vi "FPGAmain_5782_IQ_PID_Quench.vi"() -> ()   [LabVIEW 2018]
uses:
  FPGA/DataMode.ctl
  FPGA/Input_5782/5782_Fast_PID_states.ctl
  FPGA/Feed forward/FeedForwardState.ctl
  FPGA/Feed forward/FeedForwardProcessingState.ctl
  <vilib>/Platform/TimedLoop/XDataNode/timing_clust.ctl
  <vilib>/Platform/TimedLoop/XDataNode/nitl_modes.ctl
  <vilib>/Platform/TimedLoop/XDataNode/wakeup.ctl
  <vilib>/rvi/Emulation/niFpgaSctlEmulationGetInTimedLoop.vi
  <vilib>/rvi/Emulation/niFpgaEmulationReportErrorSimple.vi
  <vilib>/rvi/Emulation/niFpgaGetClockAttributes.vi
  <vilib>/rvi/Emulation/niFpgaCriticalErrorInLSC.vi
  <vilib>/rvi/Emulation/niFpgaProcessEmulError.vi
  <vilib>/rvi/Emulation/niFpgaEmulationIsFPGAContextNoSignature.vi
  <vilib>/rvi/errors/niFpgaSetErrorForExecOnDevCompSimple.vi
  <vilib>/rvi/eio/common/nirviEmuReportErrorAndStop.vi
  <vilib>/rvi/DataTransferAndStorage/Container/Common/niFpgaContainerGetUniqueNameForEmu.vi
  <vilib>/rvi/FIFO/Fifo_Resource/nirvififoEmulationSetSize.vi
  <vilib>/rvi/FIFO/Fifo_Resource/nirviFifoEmulationQueueMgr.vi
  <instcachedir>/0/nirviFifoEmulationQueueMgr_E5CAEC123FF24DC58D834DCA3CDAA9B5.lvgen/nirviFifoEmulationQueueMgr_E5CAEC123FF24DC58D834DCA3CDAA9B5_015.vi
  <vilib>/rvi/FIFO/Fifo_Resource/nirvififoEmulationDetermineInputValidOut.vi
  <vilib>/rvi/FIFO/Fifo_Resource/nirvififoEmulationCreateLock.vi
  <vilib>/rvi/FIFO/Fifo_Resource/nirvififoEmulationObtainLock.vi
  <vilib>/rvi/FIFO/Fifo_Resource/nirvififoEmulationReleaseLock.vi
  <vilib>/rvi/occurrence/nirviWaitOnOccurrenceBase.vi
  <vilib>/rvi/errors/nirviReportUnexpectedCaseInternalError.vi
  <vilib>/rvi/errors/nirviReportUnexpectedCaseInternalError (U32).vi
  <vilib>/rvi/Memory/Memory_Emulation/niFpgaMemoryEmulationCacheClearOnFirstRun.vi
  <vilib>/rvi/Memory/Memory_Emulation/nirvimemoryEmulationManagerCache_MakeExclusive.vi
  <vilib>/rvi/Memory/Memory_Emulation/niFpgaMemoryEmulationValidateCache.vi
  <vilib>/rvi/Memory/Memory_Emulation/nirvimemoryEmulationManagerCache_InsertValue.vi
  <vilib>/Utility/error.llb/Clear Errors.vi
  <vilib>/rvi/Memory/Memory_Emulation/nirvimemoryEmulationManagerCache_ReleaseExclusive.vi
  <vilib>/rvi/Memory/Memory_Emulation/nirvimemoryEmulationManagerCache_GetValue.vi
  <vilib>/rvi/Memory/Memory_Emulation/nirvimemoryEmulationManagerCache_SetValue.vi
  <vilib>/rvi/eio/common/nirviEmuTemplateMethod_errors.vi
  <instcachedir>/0/nirviFifoEmulationQueueMgr_E5CAEC123FF24DC58D834DCA3CDAA9B5.lvgen/nirviFifoEmulationQueueMgr_E5CAEC123FF24DC58D834DCA3CDAA9B5_018.vi
  <vilib>/rvi/interface/RandomDataEmulation/niFpgaRandomDataHandleErrors.vi
  <instcachedir>/0/nirviFifoEmulationQueueMgr_E5CAEC123FF24DC58D834DCA3CDAA9B5.lvgen/nirviFifoEmulationQueueMgr_E5CAEC123FF24DC58D834DCA3CDAA9B5_003.vi
  <instcachedir>/0/nirviFifoEmulationQueueMgr_E5CAEC123FF24DC58D834DCA3CDAA9B5.lvgen/nirviFifoEmulationQueueMgr_E5CAEC123FF24DC58D834DCA3CDAA9B5_017.vi
  <vilib>/rvi/interface/RandomDataEmulation/nirviRandomDataMultiElementFPGAFIFO.vi
  <instcachedir>/0/nirviRandomDataMultiElementFPGAFIFO_6740B454F3C245F78F76ED91F73FD8DB.lvgen/nirviRandomDataMultiElementFPGAFIFO_6740B454F3C245F78F76ED91F73FD8DB_000.vi
  <instrlib>/_niInstr/Basic Elements/v1/FPGA/Private/Count Down U8.vi
  <vilib>/rvi/Memory/Memory_Emulation/nirvimemoryFastEmulation.vi
  <vilib>/rvi/Memory/Memory_Emulation/nirvimemoryEmulation.vi
  <instcachedir>/0/nirviFifoEmulationQueueMgr_E5CAEC123FF24DC58D834DCA3CDAA9B5.lvgen/nirviFifoEmulationQueueMgr_E5CAEC123FF24DC58D834DCA3CDAA9B5_020.vi
  <vilib>/Platform/TimedLoop/XDataNode/XDataNode.xnode
  <vilib>/rvi/FXPMathLib/FxpInterpret/XNode/nifxpmath_Interpret.xnode
  <vilib>/rvi/DataTransferAndStorage/Container/XNode/niFpgaContainer.xnode
  <vilib>/rvi/FIFO/Fifo_Resource/nirvififoEmulationWrite.vi
  <vilib>/rvi/DataTransferAndStorage/Register/Emulation/niFpgaRegisterEmulation.vi
  <vilib>/eio/EIONode/EIONode.xnode
  <vilib>/rvi/FIFO/Fifo_Resource/nirvififoEmulationRead.vi
  <vilib>/rvi/interface/RandomDataEmulation/nirviRandomDataFpgaReadWriteTemplate.vi
  <vilib>/rvi/interface/RandomDataEmulation/nirviRandomDataFpgaMultiElementTemplate.vi
  <vilib>/Platform/TimedLoop/XDataNode/XDNodeRunTimeDep.lvlib
  <instrlib>/_niInstr/Basic Elements/v1/FPGA/niInstr Basic Elements v1 FPGA.lvlib
panel:
  out "TaM":fxp<+/-,32,13>
  out "Quench_Warning":bool
  out "Tau_set":fxp<+/-,32,13>
  in  "Ultra low speed transfer":bool
  out "5782 states":T1
  out "Read FF address":u32
  in  "Load FF":bool
  in  "Clear feedback buffers":bool
  in  "FF buffers manual":bool
  in  "Full speed transfer":bool
  in  "IO Module\\AO Data Sync":bool=TRUE
  in  "IO Module\\SPI Write Data":u16
  out "IO Module\\SPI Read Data":u8
  in  "IO Module\\SPI Read":bool
  in  "IO Module\\SPI Write":bool
  in  "IO Module\\SPI Address":u16
  in  "IO Module\\SPI Device":u8
  out "IO Module\\SPI Idle":bool
  in  "AM phase":fxp<+,64,64>
  in  "User Command Commit":bool
  in  "User Command":u8
  out "User Command Idle":bool
  out "User Command Status":u8
  in  "User Data 0":u8
  in  "User Data 1":u8
  out "PLL Locked":bool
  out "User Error":bool
  out "Configured?":bool
  in  "Continuous":bool
  in  "Record length":u16=4000 caption="Samples Per Trigger" min=1 step=1
  in  "Trigger Acquisition":bool
  out "IO Module\\Trigger Input":bool
  in  "Acquisition running":bool
  in  "Phase output":fxp<+,64,64>[](array[numeric])=[0.0, 0.0, 0.0, 0.0]
  in  "Simulated phase":fxp<+,64,64>[](array[numeric])=[0.0, 0.0]
  in  "Mode":T2
  in  "Phase input":fxp<+,64,64>[](array[numeric])=[0.0, 0.0, 0.0, 0.0, 0.0, 0.0, 0.0, 0.0, 0.0, 0.0, 0.0, 0.0, 0.0, 0.0, 0.0, 0.0]
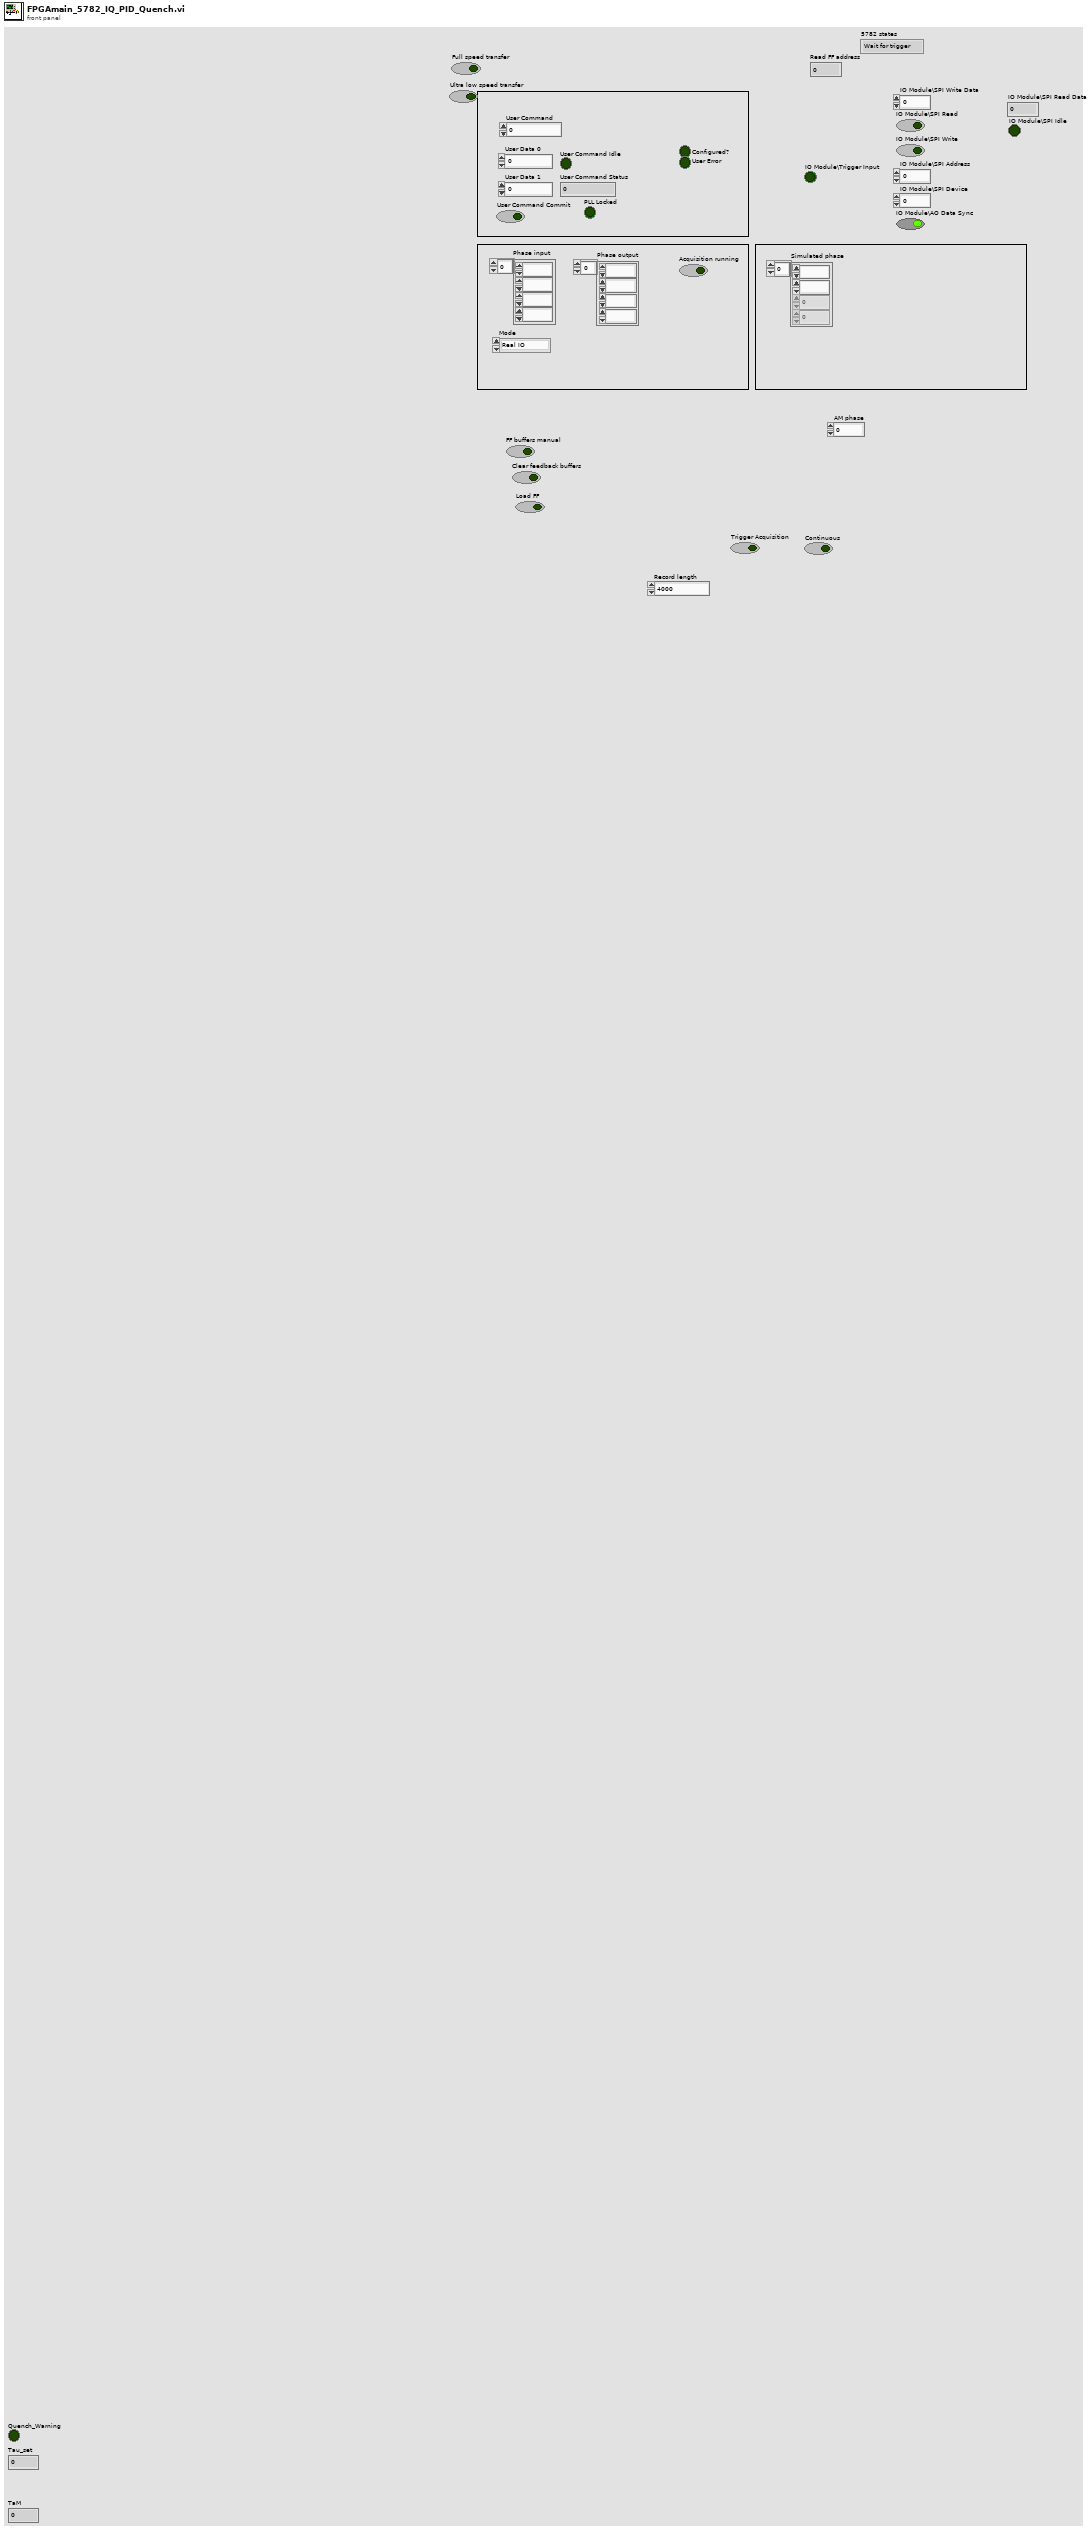
[diagram p1: front panel]
types:
  T1 = typedef "5782_Fast_PID_states.ctl" = enum8{"Wait for trigger", "Acquisition", "Send record length", "Wait for output", "Quiet period"}
  T2 = typedef "DataMode.ctl" = enum16{"Real IO", "Simulated"}
  T3 = typedef "FeedForwardProcessingState.ctl" = enum16{"Wait for trigger", "Processing", "Filtering", "Wait for reset"}
  T4 = typedef "FeedForwardState.ctl" = enum16{"Idle", "Wait for trigger", "Read FF", "Clear FF", "Wait for reset"}
  T5 = typedef "XDNodeRunTimeDep.lvlib/timing_clust.ctl" = cluster{"Expected End [f-1]":u64, "Actual End [f-1]":u64, "Finished Late? [f-1]":bool, "Expected End [i-1]":u64, "Actual End [i-1]":u64, "Finished Late? [i-1]":bool, "Expected Start [i]":u64, "Actual Start [i]":u64, "Expected Start [f]":u64, "Actual Start [f]":u64, "Source Name":string, "Structure Name":string, "Period":i64, "Deadline":i64, "Offset":i64, "Start":i64, "Priority":i32, "Timeout":i32, "Mode":T6, "Wakeup Reason":T7, "Error":errorcluster, "Source Type":string, "Secondary Source Type":string, "Global End Time":u64, "Global Start Time":u64, "Frame Duration":u64, "Iteration Duration":u64, "Assigned CPU":i32, "I/O Scan Engine Mode":u32}
  T6 = typedef "XDNodeRunTimeDep.lvlib/nitl_modes.ctl" = enum32{"No Change", "Process missed periods, maintain original phase", "Discard missed periods, maintain original phase", "Process missed periods, ignore original phase", "Discard missed periods, ignore original phase"}
  T7 = typedef "XDNodeRunTimeDep.lvlib/wakeup.ctl" = enum32{"Normal", "Aborted", "Asynchronous wakeup", "Timing source error", "Timed loop error", "Timeout"}
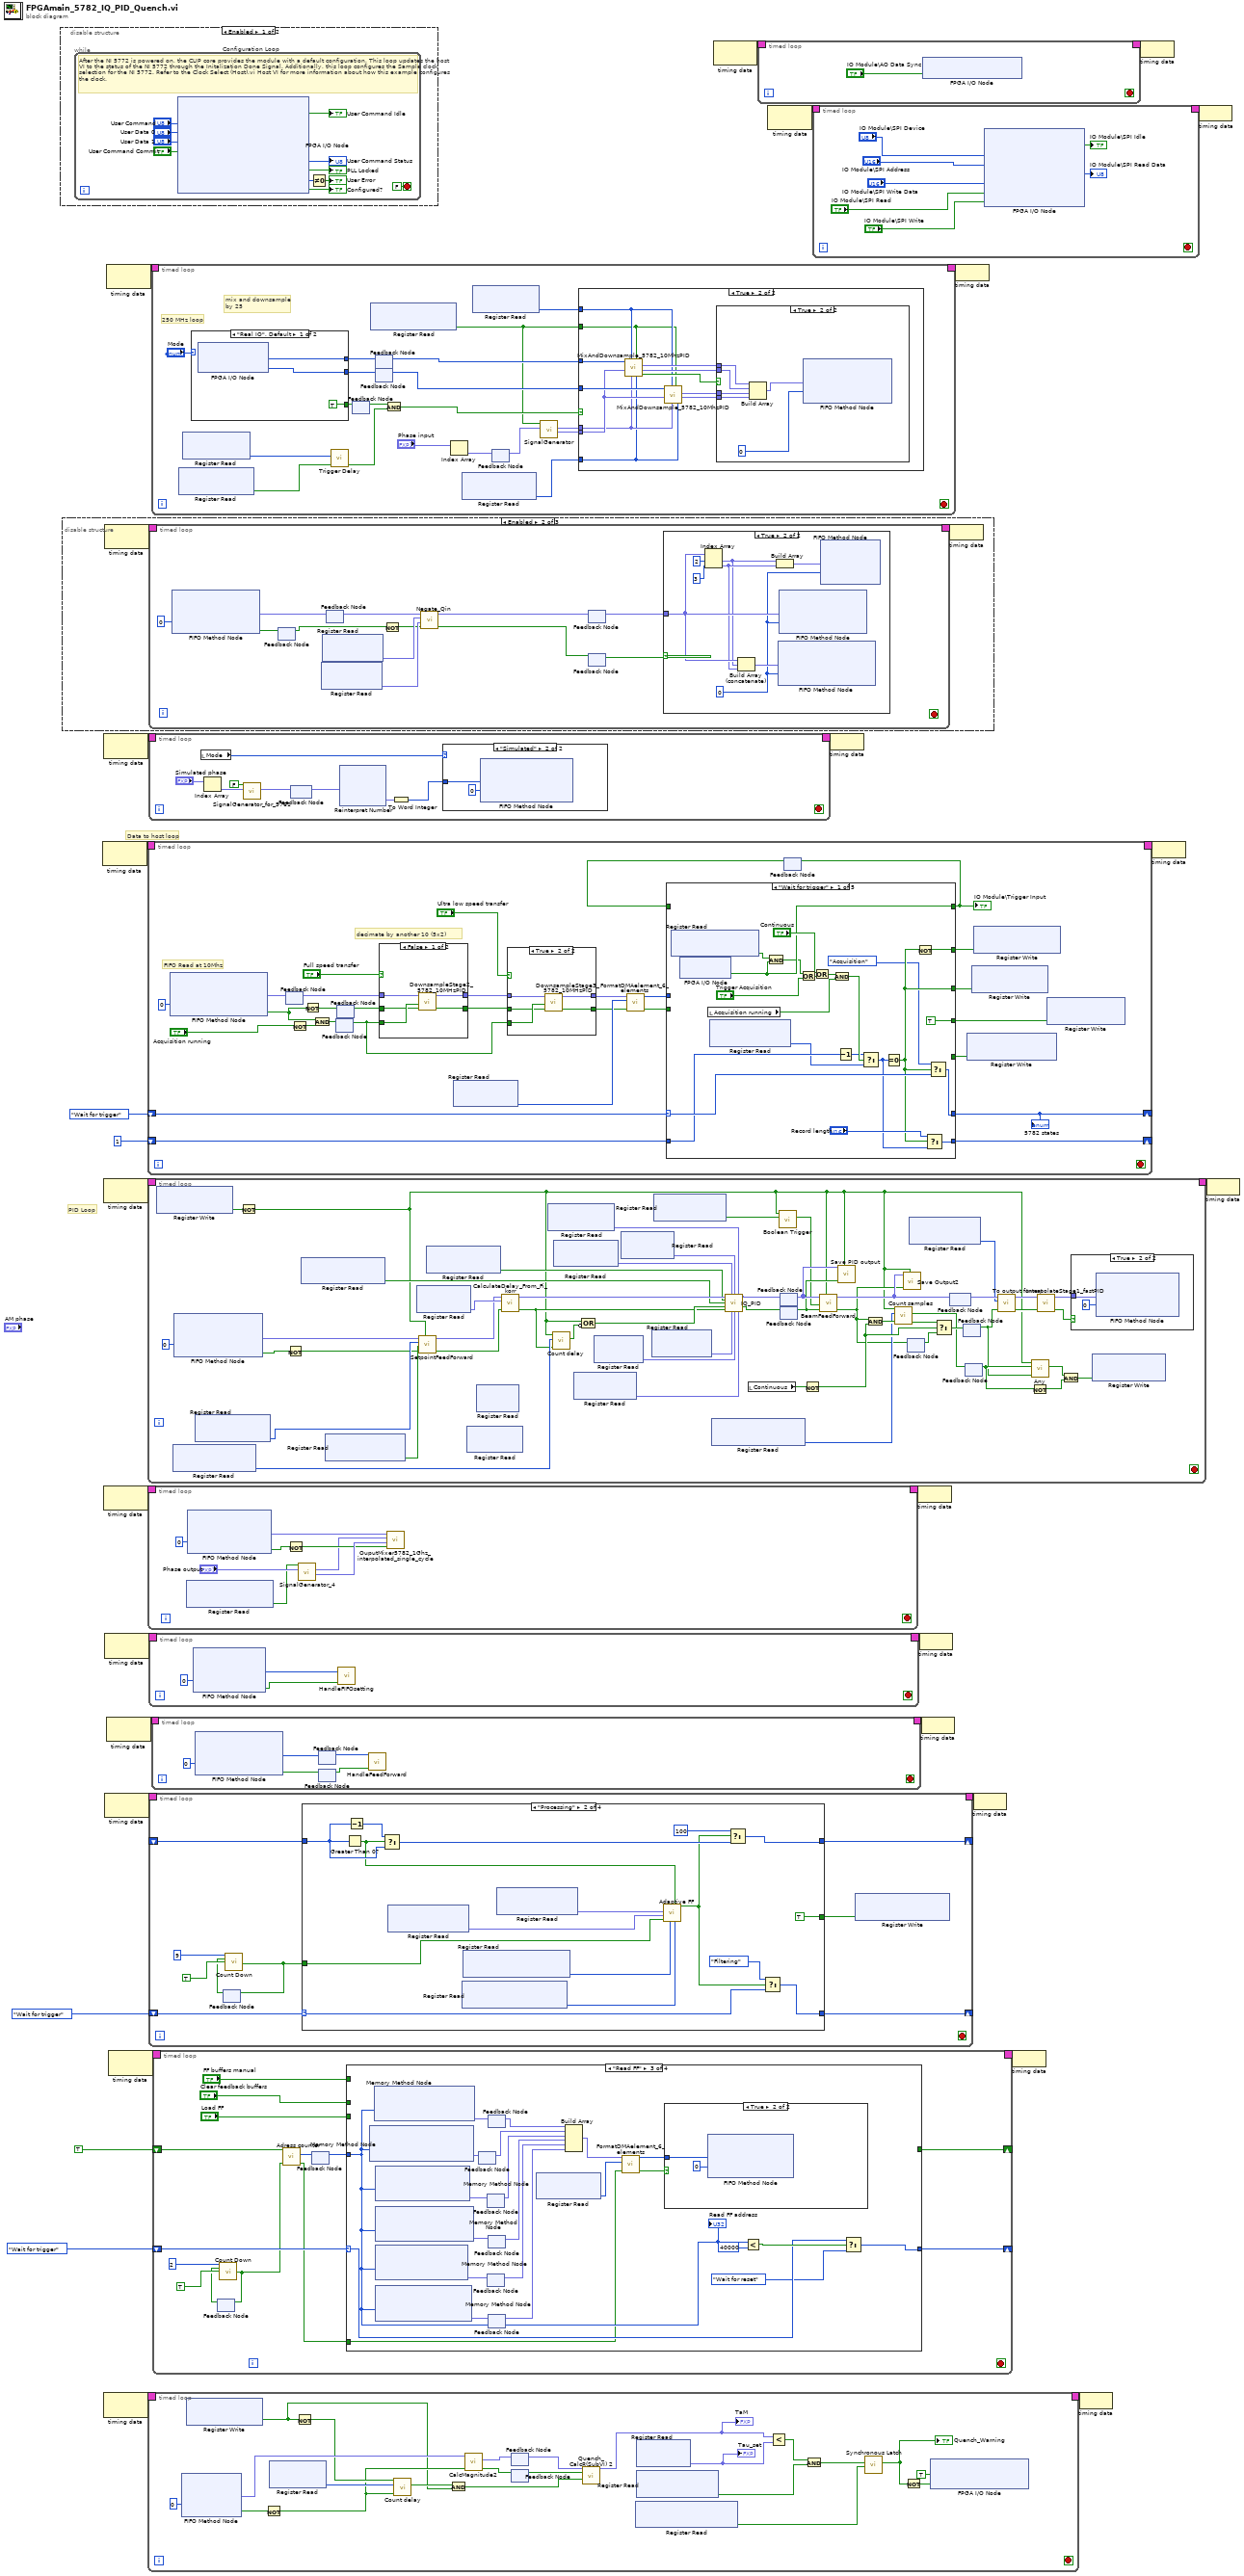
[diagram p0: block diagram]
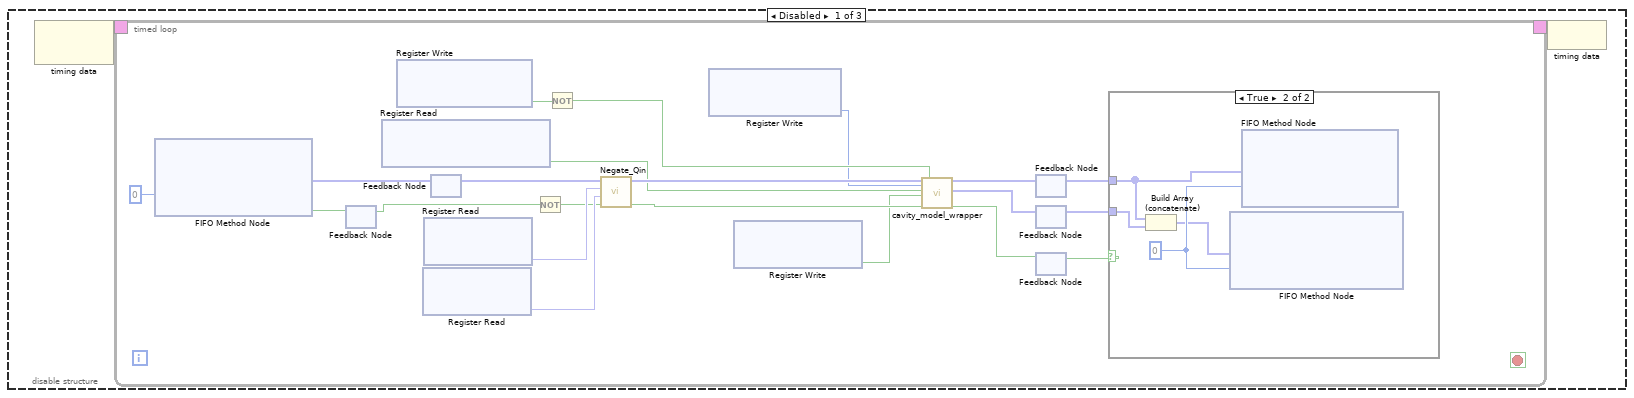
[diagram p2: hidden frame]
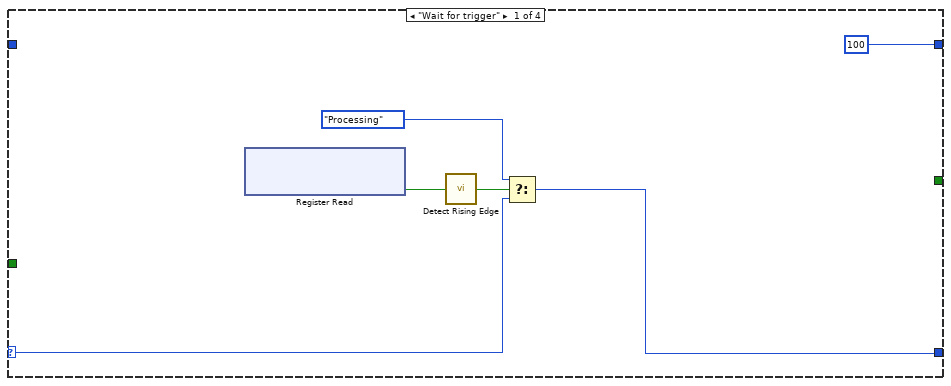
[diagram p6: hidden frame]
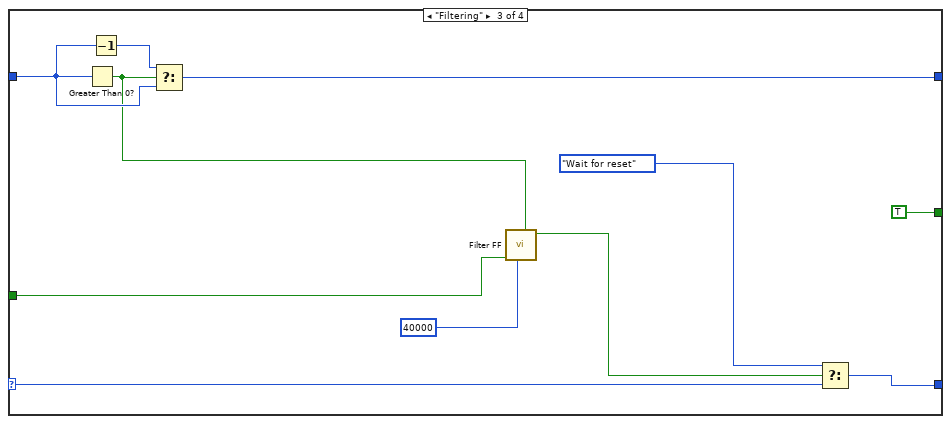
[diagram p7: hidden frame]
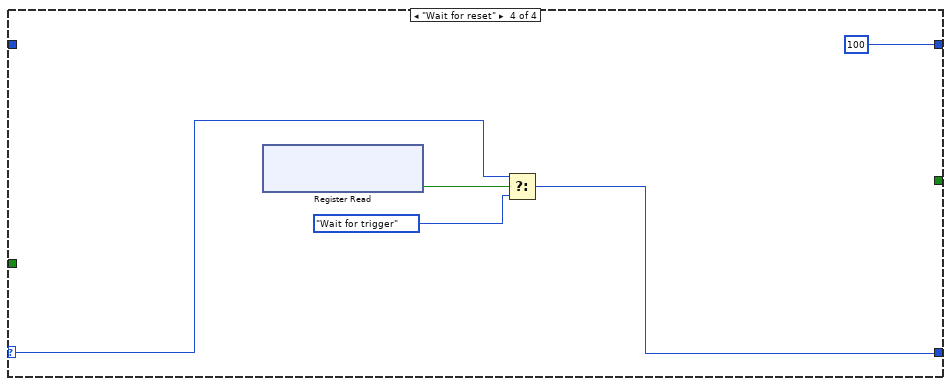
[diagram p8: hidden frame]
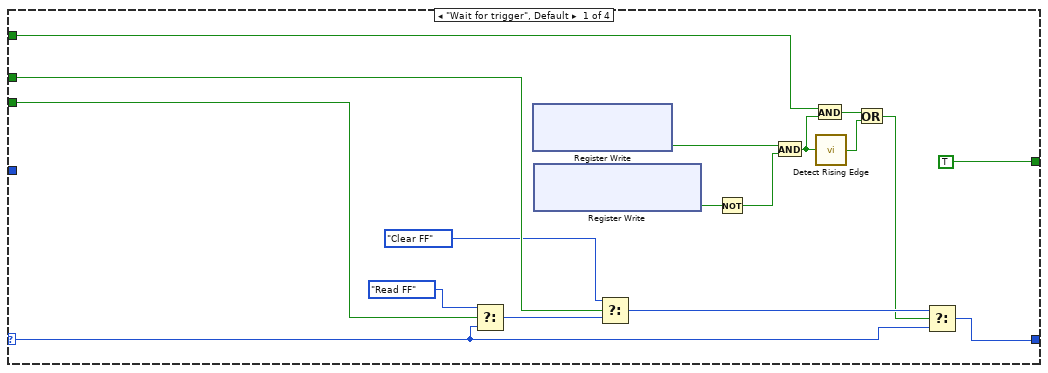
[diagram p9: hidden frame]
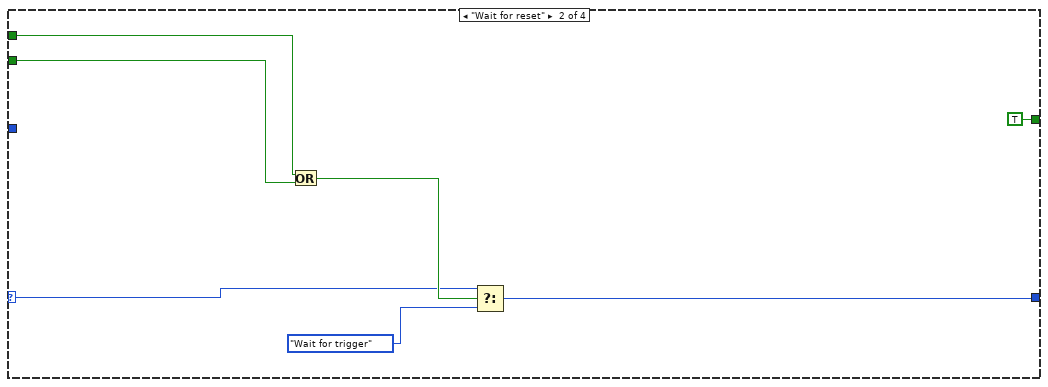
[diagram p10: hidden frame]
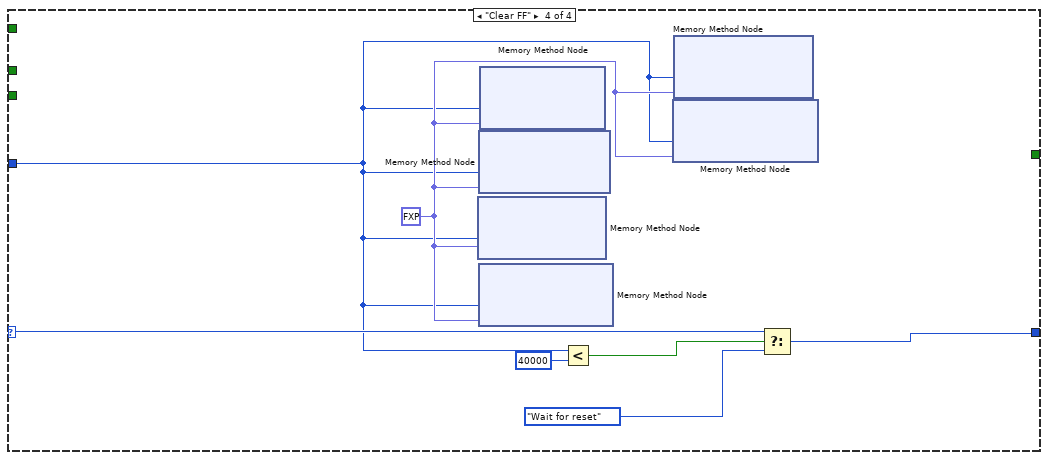
[diagram p12: hidden frame]
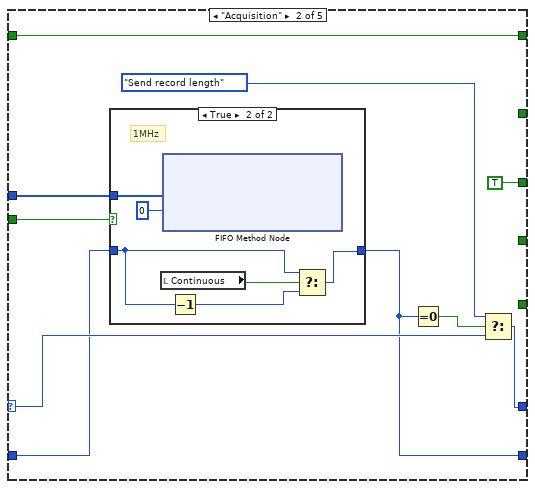
[diagram p15: hidden frame]
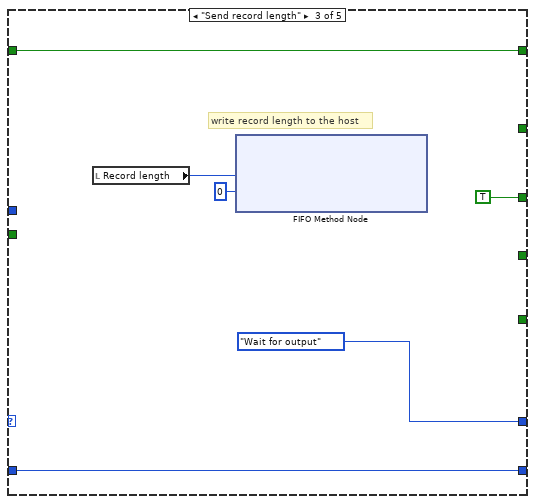
[diagram p17: hidden frame]
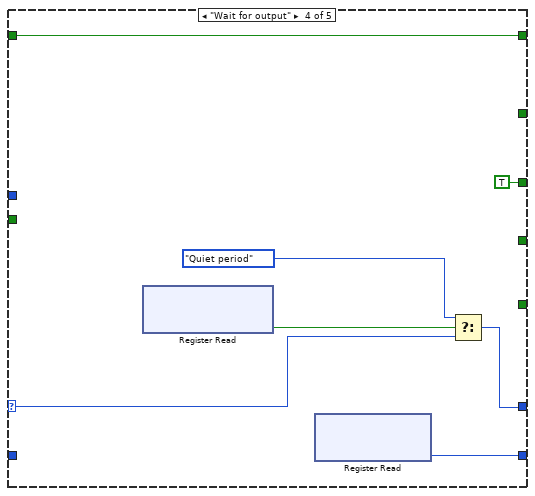
[diagram p18: hidden frame]
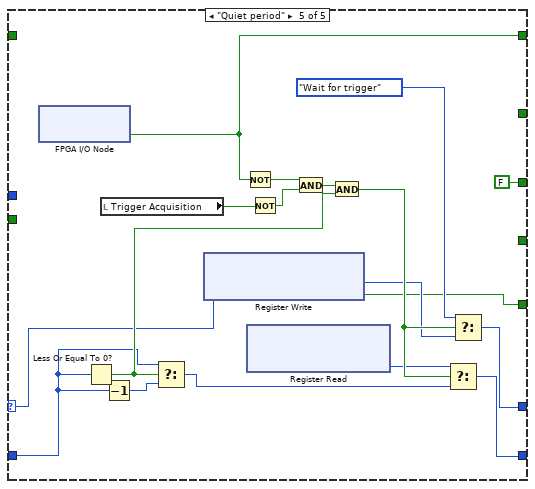
[diagram p19: hidden frame]
diagram:
  # "PID Loop"
  # "Data to host loop"
  n1 = disable-structure shown="Enabled" {
    frame Enabled {
      n2 = while "Configuration Loop" {
        stop <- FALSE stop-if-true
        # "After the NI 5772 is powered on, the CLIP core provides the module with a default configuration. This loop updates the host VI to the status of the NI 5772 through the Initalization Done Signal. Additionally, this loop configures the Sample clock selection for the NI 5772. Refer to the Clock Select (Host).vi Host VI for more information about how this example configures the clock."
        n3 = xnode "FPGA I/O Node"("IO Module\\User Command"="User Command", "IO Module\\User Data 0"="User Data 0", "IO Module\\User Data 1"="User Data 1", "IO Module\\User Command Commit"="User Command Commit") -> ("IO Module\\User Command Idle"=→"User Command Idle":bool, "IO Module\\User Command Status"=→"User Command Status":u8, "IO Module\\PLL Locked"=→"PLL Locked":bool, "IO Module\\User Error"=w35:u8, "IO Module\\Initialization Done"=→"Configured?":bool)  [unwired: 9 in, 9 out]
        n4 = Not Equal To 0?(x=w35) -> (x != 0?=→"User Error":bool)
      }
    }
    frame Disabled {
    }
  }
  n5 = disable-structure shown="Enabled" {
    frame Disabled {
      n6 = node-c288() -> (w42:T5)  [unwired: 1 in]
      n7 = timed-loop {
        timing: w42 -> [_]
        timing-out: [_] -> w41
        stop <- _ stop-if-true
        n8 = xnode ("FIFO Method Node")("Timeout"=0) -> ("Element"=w49:fxp<+/-,32,14>[], "Timed Out?"=w48:bool)  [unwired: 1 in, 1 out]
        n9 = feedback #1() -> (w46:bool)  [unwired: 1 in]
        n10 = feedback-in #1(w48) -> ()
        n11 = xnode ("Register Read")() -> ("Data"=w57:bool)  [unwired: 1 in, 1 out]
        n12 = xnode ("Register Write")() -> ("Data"=w56:bool)  [unwired: 1 in, 1 out]
        n13 = xnode ("Register Read")() -> ("Data"=w62:fxp<+/-,32,14>)  [unwired: 1 in, 1 out]
        n14 = xnode ("Register Read")() -> ("Data"=w63:fxp<+/-,32,14>)  [unwired: 1 in, 1 out]
        n15 = feedback #2() -> (w47:fxp<+/-,32,14>[])  [unwired: 1 in]
        n16 = feedback-in #2(w49) -> ()
        n17 = Not(x=w46) -> (.not. x?=w61:bool)
        n18 = Not(x=w56) -> (.not. x?=w58:bool)
        n19 = call "Negate_Qin.vi"("valid in"=w61, "DC offset chan 1"=w62, "DC offset chan 0"=w63, "Data in"=w47) -> ("valid out"=w59:bool, "Data out"=w60:fxp<+/-,32,14>[])  [unwired: 6 in]
        n20 = xnode "Register Write"() -> ("Data"=w43:enum16{"Off", "On - Ch 0", "On - Ch 1"})  [unwired: 1 in, 1 out]
        n21 = xnode "Register Write"() -> ("Data"=w44:bool)  [unwired: 1 in, 1 out]
        n22 = call "cavity_model_wrapper.vi"("Data in"=w60, "Piezo setting"=w43, "enabled"=w57, "virtual cavity"=w44, "input valid"=w59, "reset"=w58) -> ("Data out"=w55:fxp<+/-,32,14>[], "Ai1 out"=w51:fxp<+/-,32,14>[], "output valid"=w53:bool)  [unwired: 11 in]
        n23 = feedback #3() -> (w54:fxp<+/-,32,14>[])  [unwired: 1 in]
        n24 = feedback-in #3(w55) -> ()
        n25 = feedback #4() -> (w50:fxp<+/-,32,14>[])  [unwired: 1 in]
        n26 = feedback-in #4(w51) -> ()
        n27 = feedback #5() -> (w52:bool)  [unwired: 1 in]
        n28 = feedback-in #5(w53) -> ()
        n29 = case shown="True" w52 {
          tunnel: w54 -> [_ w66]
          tunnel: w50 -> [_ w65]
          frame False {
          }
          frame True {
            w67 = 0 ("Timeout")
            n30 = Build Array (concatenate)(w66, w65) -> (w64:fxp<+/-,32,14>[])
            n31 = xnode ("FIFO Method Node")("Element"=w64, "Timeout"=w67) -> ()  [unwired: 1 in, 2 out]
            n32 = xnode ("FIFO Method Node")("Element"=w66, "Timeout"=w67) -> ()  [unwired: 1 in, 2 out]
          }
        }
      }
      n33 = node-c288(w41) -> ()
    }
    frame Enabled {
      n34 = node-c288() -> (w73:T5)  [unwired: 1 in]
      n35 = timed-loop {
        timing: w73 -> [_]
        timing-out: [_] -> w72
        stop <- _ stop-if-true
        n36 = xnode ("FIFO Method Node")("Timeout"=0) -> ("Element"=w80:fxp<+/-,32,14>[], "Timed Out?"=w79:bool)  [unwired: 1 in, 1 out]
        n37 = feedback #6() -> (w77:bool)  [unwired: 1 in]
        n38 = feedback-in #6(w79) -> ()
        n39 = xnode ("Register Read")() -> ("Data"=w84:fxp<+/-,32,14>)  [unwired: 1 in, 1 out]
        n40 = xnode ("Register Read")() -> ("Data"=w85:fxp<+/-,32,14>)  [unwired: 1 in, 1 out]
        n41 = feedback #7() -> (w78:fxp<+/-,32,14>[])  [unwired: 1 in]
        n42 = feedback-in #7(w80) -> ()
        n43 = Not(x=w77) -> (.not. x?=w83:bool)
        n44 = call "Negate_Qin.vi"("valid in"=w83, "DC offset chan 1"=w84, "DC offset chan 0"=w85, "Data in"=w78) -> ("valid out"=w74:bool, "Data out"=w75:fxp<+/-,32,14>[])  [unwired: 6 in]
        n45 = feedback #8() -> (w82:fxp<+/-,32,14>[])  [unwired: 1 in]
        n46 = feedback-in #8(w75) -> ()
        n47 = feedback #9() -> (w81:bool)  [unwired: 1 in]
        n48 = feedback-in #9(w74) -> ()
        n49 = case shown="True" w81 {
          tunnel: w82 -> [_ w91]
          frame False {
          }
          frame True {
            w88 = 0 ("Timeout")
            n50 = Index Array(array=w91, index #1=2 ("index"), index #2=3 ("index")) -> (element #1=w86:fxp<+/-,32,14>, element #2=w87:fxp<+/-,32,14>)
            n51 = Build Array (concatenate)(w91, w86, w87) -> (w93:fxp<+/-,32,14>[])
            n52 = Build Array(w86, w87) -> (w92:fxp<+/-,32,14>[])
            n53 = xnode ("FIFO Method Node")("Element"=w93, "Timeout"=w88) -> ()  [unwired: 1 in, 2 out]
            n54 = xnode ("FIFO Method Node")("Element"=w91, "Timeout"=w88) -> ()  [unwired: 1 in, 2 out]
            n55 = xnode ("FIFO Method Node")("Element"=w92, "Timeout"=w88) -> ()  [unwired: 1 in, 2 out]
          }
        }
      }
      n56 = node-c288(w72) -> ()
    }
    frame Disabled {
    }
  }
  n57 = node-c288() -> (w14:T5)  [unwired: 1 in]
  n58 = node-c288() -> (w16:T5)  [unwired: 1 in]
  n59 = node-c288() -> (w22:T5)  [unwired: 1 in]
  n60 = node-c288() -> (w2:T5)  [unwired: 1 in]
  n61 = node-c288() -> (w29:T5)  [unwired: 1 in]
  n62 = node-c288() -> (w24:T5)  [unwired: 1 in]
  n63 = node-c288() -> (w5:T5)  [unwired: 1 in]
  n64 = node-c288() -> (w27:T5)  [unwired: 1 in]
  n65 = node-c288() -> (w11:T5)  [unwired: 1 in]
  n66 = node-c288() -> (w9:T5)  [unwired: 1 in]
  n67 = timed-loop {
    timing: w14 -> [_]
    timing-out: [_] -> w13
    shift-right: [w124] -> _
    shift-left: 5782_Fast_PID_states."Wait for trigger" ("5782 states") -> [w126]
    shift-right: [w123] -> _
    shift-left: u16 1 ("trigger samples") -> [w125]
    stop <- _ stop-if-true
    # "FIFO Read at 10Mhz"
    # "decimate by another 10 (5x2)"
    n68 = xnode ("FIFO Method Node")("Timeout"=0) -> ("Element"=w106:fxp<+/-,32,14>[], "Timed Out?"=w105:bool)  [unwired: 1 in, 1 out]
    n69 = feedback #10() -> (w107:fxp<+/-,32,14>[])  [unwired: 1 in]
    n70 = feedback-in #10(w106) -> ()
    n71 = Not(x="Acquisition running") -> (.not. x?=w112:bool)
    n72 = Not(x=w105) -> (.not. x?=w110:bool)
    n73 = And(x=w105, y=w112) -> (x .and. y?=w109:bool)
    n74 = feedback #11() -> (w102:bool)  [unwired: 1 in]
    n75 = feedback-in #11(w109) -> ()
    n76 = feedback #12() -> (w111:bool)  [unwired: 1 in]
    n77 = feedback-in #12(w110) -> ()
    n78 = case shown="False" "Full speed transfer" {
      tunnel: [w138 w140] -> w100
      tunnel: [w137 w139] -> w101
      tunnel: w107 -> [w136 w140]
      tunnel: w102 -> [w135 _]
      tunnel: w111 -> [w134 w139]
      frame False {
        n79 = call "DownsampleStage2_5782_10MHzPID.vi"("valid in"=w134, "reset"=w135, "Data in"=w136) -> ("valid out"=w137:bool, "data out"=w138:fxp<+/-,32,14>[])  [unwired: 7 in]
      }
      frame True {
      }
    }
    n80 = xnode ("Register Read")() -> ("Data"=w116:u16)  [unwired: 1 in, 1 out]
    n81 = case shown="True" "Ultra low speed transfer" {
      tunnel: [w128 w132] -> w98
      tunnel: [w127 w131] -> w99
      tunnel: w100 -> [w128 w133]
      tunnel: w102 -> [_ w130]
      tunnel: w101 -> [w127 w129]
      frame False {
      }
      frame True {
        n82 = call "DownsampleStage3_5782_10MHzPID.vi"("valid in"=w129, "reset"=w130, "Data in"=w133) -> ("valid out"=w131:bool, "data out"=w132:fxp<+/-,32,14>[])  [unwired: 7 in]
      }
    }
    n83 = call "FormatDMAelement_6_elements.vi"("valid in"=w99, "factor"=w116, "Data in"=w98) -> ("valid out"=w119:bool, "Values"=w118:u64[])  [unwired: 7 in]
    n84 = feedback #13() -> (w121:bool)  [unwired: 1 in]
    n85 = case shown="\"Wait for trigger\"" w126 {
      selector: w126 -> [w161 w171 _ w189 w196]
      tunnel: w125 -> [w152 w168 w179 _ w197]
      tunnel: [w160 w170 5782_Fast_PID_states."Wait for output" ("5782 states") w191 w207] -> w124
      tunnel: [w159 w165 w179 w187 w208] -> w123
      tunnel: w118 -> [_ w166 _ _ _]
      tunnel: w119 -> [_ w167 _ _ _]
      tunnel: [w147 TRUE TRUE ("5782 triggered") TRUE ("5782 triggered") FALSE ("5782 triggered")] -> w122
      tunnel: [w142 w164 w181 w186 w192] -> w120
      tunnel: w121 -> [_ w164 w181 w186 _]
      tunnel: [w146 _ _ _ _] -> w117
      tunnel: [TRUE _ _ _ _] -> w115
      tunnel: [_ _ _ _ w194] -> w114
      frame "Wait for trigger" {
        n86 = xnode ("Register Read")() -> ("Data"=w143:bool)  [unwired: 1 in, 1 out]
        n87 = xnode "FPGA I/O Node"() -> ("PXI_Trig0"=w142:bool)  [unwired: 1 in, 1 out]
        n88 = local read "Acquisition running"() -> (w155:bool)
        n89 = xnode ("Register Read")() -> ("Data"=w148:u16)  [unwired: 1 in, 1 out]
        n90 = And(x=w143, y=w142) -> (x .and. y?=w141:bool)
        n91 = Or(x=w141, y="Trigger Acquisition") -> (x .or. y?=w151:bool)
        n92 = Or(x="Continuous", y=w151) -> (x .or. y?=w149:bool)
        n93 = And(x=w149, y=w155) -> (x .and. y?=w156:bool)
        n94 = Decrement(x=w152) -> (x-1=w153:u16)
        n95 = Select(t=w153, s=w156, f=w148) -> (s? t:f=w154:u16)
        n96 = Equal To 0?(x=w154) -> (x = 0?=w147:bool)
        n97 = Not(x=w147) -> (.not. x?=w146:bool)
        n98 = Select(t="Record length", s=w147, f=w154) -> (s? t:f=w159:u16)
        n99 = Select(t=5782_Fast_PID_states."Acquisition" ("5782 states"), s=w147, f=w161) -> (s? t:f=w160:T1)
      }
      frame "Acquisition" {
        n100 = case shown="True" w167 {
          tunnel: w166 -> [_ w178]
          tunnel: [w172 w175] -> w165
          tunnel: w168 -> [w172 w173]
          frame False {
          }
          frame True {
            # "1MHz"
            n101 = local read "Continuous"() -> (w176:bool)
            n102 = xnode ("FIFO Method Node")("Element"=w178, "Timeout"=0) -> ()  [unwired: 1 in, 2 out]
            n103 = Decrement(x=w173) -> (x-1=w174:u16)
            n104 = Select(t=w173, s=w176, f=w174) -> (s? t:f=w175:u16)
          }
        }
        n105 = Equal To 0?(x=w165) -> (x = 0?=w169:bool)
        n106 = Select(t=5782_Fast_PID_states."Send record length" ("5782 states"), s=w169, f=w171) -> (s? t:f=w170:T1)
      }
      frame "Send record length" {
        # "write record length to the host"
        n107 = local read "Record length"() -> (w183:u16)
        n108 = xnode ("FIFO Method Node")("Element"=w183, "Timeout"=0) -> ()  [unwired: 1 in, 2 out]
      }
      frame "Wait for output" {
        n109 = xnode ("Register Read")() -> ("Data"=w185:bool)  [unwired: 1 in, 1 out]
        n110 = xnode ("Register Read")() -> ("Data"=w187:u16)  [unwired: 1 in, 1 out]
        n111 = Select(t=5782_Fast_PID_states."Quiet period" ("5782 states"), s=w185, f=w189) -> (s? t:f=w191:T1)
      }
      frame "Quiet period" {
        n112 = xnode "FPGA I/O Node"() -> ("PXI_Trig0"=w192:bool)  [unwired: 1 in, 1 out]
        n113 = Less Or Equal To 0?(x=w197) -> (x <= 0?=w200:bool)
        n114 = local read "Trigger Acquisition"() -> (w205:bool)
        n115 = Decrement(x=w197) -> (x-1=w201:u16)
        n116 = Select(t=w197, s=w200, f=w201) -> (s? t:f=w199:u16)
        n117 = xnode ("Register Write")() -> ("Data"=w194:bool)  [unwired: 1 in, 1 out]
        n118 = Not(x=w192) -> (.not. x?=w193:bool)
        n119 = xnode ("Register Read")() -> ("Data"=w198:u16)  [unwired: 1 in, 1 out]
        n120 = Not(x=w205) -> (.not. x?=w204:bool)
        n121 = And(x=w193, y=w204) -> (x .and. y?=w203:bool)
        n122 = And(x=w203, y=w200) -> (x .and. y?=w206:bool)
        n123 = Select(t=w198, s=w206, f=w199) -> (s? t:f=w208:u16)
        n124 = Select(t=5782_Fast_PID_states."Wait for trigger" ("5782 states"), s=w206, f=w196) -> (s? t:f=w207:T1)
      }
    }
    "IO Module\\Trigger Input" <- w120
    "5782 states" <- w124
    n125 = feedback-in #13(w120) -> ()
    n126 = xnode ("Register Write")("Data"=w114) -> ()  [unwired: 1 in, 1 out]
    n127 = xnode ("Register Write")("Data"=w122) -> ()  [unwired: 1 in, 1 out]
    n128 = xnode ("Register Write")("Data"=w117) -> ()  [unwired: 1 in, 1 out]
    n129 = xnode ("Register Write")("Data"=w115) -> ()  [unwired: 1 in, 1 out]
  }
  n130 = timed-loop {
    timing: w16 -> [_]
    timing-out: [_] -> w15
    stop <- _ stop-if-true
    n131 = xnode ("Register Write")() -> ("Data"=w259:bool)  [unwired: 1 in, 1 out]
    n132 = xnode ("Register Read")() -> ("Data"=w255:u32)  [unwired: 1 in, 1 out]
    n133 = xnode ("FIFO Method Node")("Timeout"=0) -> ("Element"=w253:fxp<+/-,32,14>[], "Timed Out?"=w260:bool)  [unwired: 1 in, 1 out]
    n134 = xnode ("Register Read")() -> ("Data"=w254:u32)  [unwired: 1 in, 1 out]
    n135 = Not(x=w259) -> (.not. x?=w213:bool)
    n136 = Not(x=w260) -> (.not. x?=w252:bool)
    n137 = xnode ("Register Read")() -> ("Data"=w239:bool)  [unwired: 1 in, 1 out]
    n138 = xnode ("Register Read")() -> ("Data"=w258:bool)  [unwired: 1 in, 1 out]
    n139 = xnode ("Register Read")() -> ("Data"=w251:fxp<+/-,32,4>)  [unwired: 1 in, 1 out]
    n140 = call "SetpointFeedForward.vi"("Reset"=w213, "input valid"=w252, "setpoint enabled"=w258, "Samples to skip"=w254, "Data in"=w253) -> ("output valid"=w250:bool, "Data out"=w249:fxp<+/-,32,14>[])  [unwired: 5 in]
    n141 = xnode ("Register Read")() -> ("Data"=w247:bool)  [unwired: 1 in, 1 out]
    n142 = xnode ("Register Read")() -> ()  [unwired: 1 in, 2 out]
    n143 = xnode ("Register Read")() -> ()  [unwired: 1 in, 2 out]
    n144 = call "CalculateDelay_From_Fi_korr.vi"("input valid"=w250, "fi_korr"=w251, "Data in"=w249) -> ("output valid"=w240:bool, "Data out"=w248:fxp<+/-,32,14>[])  [unwired: 7 in]
    n145 = xnode ("Register Read")() -> ("Data"=w242:fxp<+/-,32,6>)  [unwired: 1 in, 1 out]
    n146 = call "Count delay.vi"("input valid"=w240, "Count to skip"=w255, "Reset"=w213) -> ("count done?"=w256:bool)  [unwired: 7 in, 1 out]
    n147 = xnode ("Register Read")() -> ("Data"=w246:fxp<+/-,32,6>)  [unwired: 1 in, 1 out]
    n148 = xnode ("Register Read")() -> ("Data"=w236:fxp<+/-,32,6>)  [unwired: 1 in, 1 out]
    n149 = Compound Arithmetic op=OR(w213, invert w256) -> (w241:bool)
    n150 = xnode ("Register Read")() -> ("Data"=w237:fxp<+/-,32,6>)  [unwired: 1 in, 1 out]
    n151 = xnode ("Register Read")() -> ("Data"=w245:fxp<+/-,32,6>)  [unwired: 1 in, 1 out]
    n152 = xnode ("Register Read")() -> ("Data"=w238:fxp<+/-,32,6>)  [unwired: 1 in, 1 out]
    n153 = xnode ("Register Read")() -> ("Data"=w214:bool)  [unwired: 1 in, 1 out]
    n154 = xnode ("Register Read")() -> ("Data"=w226:u32)  [unwired: 1 in, 1 out]
    n155 = call "IQ_PID.vi"("Data in"=w248, "Ki*Tau I"=w246, "Kp I"=w245, "Kd/Tau I"=w242, "Enable I"=w247, "Enable Q"=w239, "Reset"=w241, "input valid"=w240, "Ki*Tau Q"=w238, "Kp Q"=w237, "Kd/Tau Q"=w236) -> ("data out"=w244:fxp<+/-,32,14>[], "output valid"=w243:bool)  [unwired: 3 in]
    n156 = local read "Continuous"() -> (w235:bool)
    n157 = call "Boolean Trigger.vi"("Value"=w214, "Reset"=w213) -> ("Value out"=w212:bool)  [unwired: 9 in]
    n158 = feedback #14() -> (w218:fxp<+/-,32,14>[])  [unwired: 1 in]
    n159 = feedback-in #14(w244) -> ()
    n160 = feedback #15() -> (w217:bool)  [unwired: 1 in]
    n161 = feedback-in #15(w243) -> ()
    n162 = Not(x=w235) -> (.not. x?=w228:bool)
    n163 = call "BeamFeedForward.vi"("Reset"=w213, "input valid"=w217, "beam enabled"=w212, "Data in"=w218) -> ("output valid"=w215:bool, "Data out"=w216:fxp<+/-,32,14>[])  [unwired: 6 in]
    n164 = call "Save PID output.vi"("Reset"=w213, "input valid"=w217, "Data in"=w218) -> ()  [unwired: 9 in]
    n165 = And(x=w215, y=w228) -> (x .and. y?=w230:bool)
    n166 = call "Count samples.vi"("input valid"=w230, "number to count"=w226, "Reset"=w213) -> ("output valid"=w231:bool, "counting"=w227:bool)  [unwired: 7 in]
    n167 = call "Save Output2.vi"("Reset"=w213, "input valid"=w215, "Data in"=w216) -> ()  [unwired: 9 in]
    n168 = feedback #16() -> (w229:bool)  [unwired: 1 in]
    n169 = feedback-in #16(w215) -> ()
    n170 = xnode ("Register Read")() -> ("Data"=w219:u16)  [unwired: 1 in, 1 out]
    n171 = Select(t=w231, s=w228, f=w229) -> (s? t:f=w232:bool)
    n172 = feedback #17() -> (w223:fxp<+/-,32,14>[])  [unwired: 1 in]
    n173 = feedback-in #17(w216) -> ()
    n174 = feedback-in #18(w232) -> ()
    n175 = feedback #18() -> (w221:bool)  [unwired: 1 in]
    n176 = feedback #19() -> (w234:bool)  [unwired: 1 in]
    n177 = feedback-in #19(w227) -> ()
    n178 = call "To output format.vi"("input valid"=w221, "factor"=w219, "Data in"=w223) -> ("output valid"=w220:bool, "Data out"=w222:fxp<+/-,16,14>[])  [unwired: 7 in]
    n179 = Not(x=w234) -> (.not. x?=w233:bool)
    n180 = call "Any.vi"("input valid"=w221, "Value"=w234, "Reset"=w213) -> ("Any?"=w211:bool)  [unwired: 7 in, 1 out]
    n181 = call "InterpolateStage1_fastPID.vi"("valid in"=w220, "Data in"=w222) -> ("valid out"=w224:bool, "Data out"=w225:fxp<+/-,16,14>[])  [unwired: 8 in]
    n182 = And(x=w211, y=w233) -> (x .and. y?=w257:bool)
    n183 = case shown="True" w224 {
      tunnel: w225 -> [_ w263]
      frame False {
      }
      frame True {
        n184 = xnode ("FIFO Method Node")("Element"=w263, "Timeout"=0) -> ()  [unwired: 1 in, 2 out]
      }
    }
    n185 = xnode ("Register Write")("Data"=w257) -> ()  [unwired: 1 in, 1 out]
  }
  n186 = timed-loop {
    timing: w22 -> [_]
    timing-out: [_] -> w21
    stop <- _ stop-if-true
    n187 = xnode ("Register Read")() -> ("Data"=w266:bool)  [unwired: 1 in, 1 out]
    n188 = xnode ("FIFO Method Node")("Timeout"=0) -> ("Element"=w269:fxp<+/-,16,14>[], "Timed Out?"=w272:bool)  [unwired: 1 in, 1 out]
    n189 = Not(x=w272) -> (.not. x?=w268:bool)
    n190 = call "SignalGenerator_4.vi"("Phase"="Phase output", "reset"=w266) -> ("Sine out"=w270:fxp<+/-,16,0>[], "Cosine out"=w267:fxp<+/-,16,0>[])  [unwired: 8 in]
    n191 = call "OuputMixer5782_1Ghz_interpolated_single_cycle.vi"("input valid"=w268, "Sine in"=w270, "Cosine in"=w267, "Data"=w269) -> ()  [unwired: 7 in, 1 out]
  }
  n192 = timed-loop {
    timing: w2 -> [_]
    timing-out: [_] -> w1
    stop <- _ stop-if-true
    n193 = xnode ("FIFO Method Node")("Timeout"=0) -> ("Element"=w284:fxp<+/-,32,14>[], "Timed Out?"=w282:bool)  [unwired: 1 in, 1 out]
    n194 = xnode ("Register Write")() -> ("Data"=w278:bool)  [unwired: 1 in, 1 out]
    n195 = Not(x=w282) -> (.not. x?=w281:bool)
    n196 = xnode ("Register Read")() -> ("Data"=w285:u32)  [unwired: 1 in, 1 out]
    n197 = Not(x=w278) -> (.not. x?=w283:bool)
    n198 = call "Count delay.vi"("input valid"=w281, "Count to skip"=w285, "Reset"=w283) -> ("count done?"=w289:bool)  [unwired: 7 in, 1 out]
    n199 = And(x=w289, y=w278) -> (x .and. y?=w286:bool)
    n200 = call "CalcMagnitude2.vi"("input valid"=w281, "Data in"=w284) -> ("output valid"=w290:bool, "Amp1"=w291:fxp<+,16,14>)  [unwired: 8 in]
    n201 = feedback #20() -> (w288:fxp<+,16,14>)  [unwired: 1 in]
    n202 = feedback-in #20(w291) -> ()
    n203 = feedback #21() -> (w287:bool)  [unwired: 1 in]
    n204 = feedback-in #21(w290) -> ()
    n205 = call "Quench_CalcR(SubVI) 2.vi"("Mag"=w288, "input valid"=w287, "count done?"=w286) -> ("Tau meas"=w279:fxp<+/-,32,13>)  [unwired: 12 in]
    "TaM" <- w279
    n206 = xnode ("Register Read")() -> ("Data"=w295:bool)  [unwired: 1 in, 1 out]
    n207 = xnode ("Register Read")() -> ("Data"=w293:fxp<+/-,32,13>)  [unwired: 1 in, 1 out]
    "Tau_set" <- w293
    n208 = xnode ("Register Read")() -> ("Data"=w297:bool)  [unwired: 1 in, 1 out]
    n209 = Less?(x=w279, y=w293) -> (x < y?=w296:bool)
    n210 = And(x=w296, y=w297) -> (x .and. y?=w294:bool)
    n211 = call <instrlib>:"Synchronous Latch.vi"("clear"=w295, "set"=w294) -> ("out"=w292:bool)  [unwired: 9 in]
    "Quench_Warning" <- w292
    n212 = Not(x=w292) -> (.not. x?=w277:bool)
    n213 = xnode "FPGA I/O Node"("IO Module\\PFI 2 WE"=TRUE ("IO Module\\PFI 2 WE"), "IO Module\\PFI 2 Wr Data"=w277) -> ()  [unwired: 2 in, 2 out]
  }
  n214 = timed-loop {
    timing: w29 -> [_]
    timing-out: [_] -> w28
    stop <- _ stop-if-true
    n215 = local read "Mode"() -> (w307:T2)
    n216 = Index Array(array="Simulated phase") -> (element=w306:fxp<+,64,64>)  [unwired: 1 in]
    n217 = call "SignalGenerator_for_5761.vi"("phase"=w306, "Reset"=FALSE) -> ("Sin"=w302:fxp<+/-,16,0>)  [unwired: 7 in, 2 out]
    n218 = feedback #22() -> (w303:fxp<+/-,16,0>)  [unwired: 1 in]
    n219 = feedback-in #22(w302) -> ()
    n220 = xnode "Reinterpret Number"("x"=w303) -> ("y"=w304:fxp<+/-,16,13>)
    n221 = To Word Integer(number=w304) -> (16bit integer=w300:i16)
    n222 = case shown="\"Simulated\"" w307 {
      tunnel: w300 -> [_ w308]
      frame "Real IO", Default {
      }
      frame "Simulated" {
        n223 = xnode ("FIFO Method Node")("Element"=w308, "Timeout"=0) -> ()  [unwired: 1 in, 2 out]
      }
    }
  }
  n224 = timed-loop {
    timing: w24 -> [_]
    timing-out: [_] -> w23
    stop <- _ stop-if-true
    n225 = xnode ("FIFO Method Node")("Timeout"=0) -> ("Element"=w313:u64, "Timed Out?"=w312:bool)  [unwired: 1 in, 1 out]
    n226 = call "HandleFIFOsetting.vi"("timed out"=w312, "Value"=w313) -> ()  [unwired: 10 in]
  }
  n227 = timed-loop {
    timing: w5 -> [_]
    timing-out: [_] -> w4
    shift-right: [w320] -> _
    shift-left: FeedForwardProcessingState."Wait for trigger" ("Processing state") -> [w321]
    shift-right: [w318] -> _
    shift-left: _ -> [w319]
    stop <- _ stop-if-true
    n228 = feedback #23() -> (w323:bool)  [unwired: 1 in]
    n229 = call-poly <instrlib>:"Count Down.vi"("count in"=u8 9, "load"=w323, "decrement"=TRUE) -> ("terminal count"=w322:bool)  [unwired: 11 in, 1 out]
    n230 = feedback-in #23(w322) -> ()
    n231 = case shown="\"Processing\"" w321 {
      selector: w321 -> [w330 w338 w354 w362]
      tunnel: w322 -> [_ w334 w350 _]
      tunnel: [w329 w336 w352 w361] -> w320
      tunnel: w319 -> [_ w344 w357 _]
      tunnel: [u8 100 ("unsigned 8bit integer") w340 w348 u8 100 ("unsigned 8bit integer")] -> w318
      tunnel: [_ TRUE ("Data") TRUE ("Data") _] -> w317
      frame "Wait for trigger" {
        n232 = xnode ("Register Read")() -> ("Data"=w327:bool)  [unwired: 1 in, 1 out]
        n233 = call <instrlib>:"Detect Rising Edge.vi"("signal"=w327) -> ("edge detected"=w326:bool)  [unwired: 14 in]
        n234 = Select(t=FeedForwardProcessingState."Processing" ("Processing state"), s=w326, f=w330) -> (s? t:f=w329:T3)
      }
      frame "Processing" {
        n235 = Greater Than 0?(x=w344) -> (x > 0?=w343:bool)
        n236 = Decrement(x=w344) -> (x-1=w345:u8)
        n237 = Select(t=w345, s=w343, f=w344) -> (s? t:f=w341:u8)
        n238 = xnode ("Register Read")() -> ("Data"=w332:fxp<+/-,32,2>)  [unwired: 1 in, 1 out]
        n239 = xnode ("Register Read")() -> ("Data"=w347:u32)  [unwired: 1 in, 1 out]
        n240 = xnode ("Register Read")() -> ("Data"=w346:u32)  [unwired: 1 in, 1 out]
        n241 = xnode ("Register Read")() -> ("Data"=w333:fxp<+/-,32,2>)  [unwired: 1 in, 1 out]
        n242 = call "Adaptive FF.vi"("Source start addr"=w347, "Reset"=w343, "Destination start addr"=w346, "input valid"=w334, "a0"=w332, "b0"=w333) -> ("done"=w339:bool)  [unwired: 4 in, 1 out]
        n243 = Select(t=u8 100 ("s? t:f"), s=w339, f=w341) -> (s? t:f=w340:u8)
        n244 = Select(t=FeedForwardProcessingState."Filtering", s=w339, f=w338) -> (s? t:f=w336:T3)
      }
      frame "Filtering" {
        n245 = Greater Than 0?(x=w357) -> (x > 0?=w356:bool)
        n246 = Decrement(x=w357) -> (x-1=w358:u8)
        n247 = Select(t=w358, s=w356, f=w357) -> (s? t:f=w348:u8)
        n248 = call "Filter FF.vi"("Reset"=w356, "Elements in buffer"=u32 40000, "input valid"=w350) -> ("done"=w355:bool)  [unwired: 7 in, 1 out]
        n249 = Select(t=FeedForwardProcessingState."Wait for reset", s=w355, f=w354) -> (s? t:f=w352:T3)
      }
      frame "Wait for reset" {
        n250 = xnode ("Register Read")() -> ("Data"=w359:bool)  [unwired: 1 in, 1 out]
        n251 = Select(t=w362, s=w359, f=FeedForwardProcessingState."Wait for trigger" ("Processing state")) -> (s? t:f=w361:T3)
      }
    }
    n252 = xnode ("Register Write")("Data"=w317) -> ()  [unwired: 1 in, 1 out]
  }
  n253 = timed-loop {
    timing: w27 -> [_]
    timing-out: [_] -> w26
    stop <- _ stop-if-true
    # "mix and downsample\nby 25"
    # "250 MHz loop"
    n254 = xnode ("Register Read")() -> ("Data"=w371:bool)  [unwired: 1 in, 1 out]
    n255 = xnode ("Register Read")() -> ("Data"=w369:u32)  [unwired: 1 in, 1 out]
    n256 = case shown="\"Real IO\", Default" "Mode" {
      tunnel: [w405 w406] -> w383
      tunnel: [w404 w406] -> w381
      tunnel: [TRUE w407] -> w379
      frame "Real IO", Default {
        n257 = xnode "FPGA I/O Node"() -> ("IO Module\\AI 0"=w405:i16, "IO Module\\AI 1"=w404:i16)  [unwired: 2 in, 2 out]
      }
      frame "Simulated" {
        n258 = xnode ("FIFO Method Node")("Timeout"=0) -> ("Element"=w406:i16, "Timed Out?"=w408:bool)  [unwired: 1 in, 1 out]
        n259 = Not(x=w408) -> (.not. x?=w407:bool)
      }
    }
    n260 = call "Trigger Delay.vi"("input valid"=w371, "Count to skip"=w369) -> ("output valid"=w370:bool)  [unwired: 9 in]
    n261 = feedback #24() -> (w378:bool)  [unwired: 1 in]
    n262 = feedback-in #24(w379) -> ()
    n263 = xnode ("Register Read")() -> ("Data"=w367:bool)  [unwired: 1 in, 1 out]
    n264 = feedback #25() -> (w382:i16)  [unwired: 1 in]
    n265 = feedback-in #25(w383) -> ()
    n266 = feedback #26() -> (w380:i16)  [unwired: 1 in]
    n267 = feedback-in #26(w381) -> ()
    n268 = And(x=w378, y=w370) -> (x .and. y?=w375:bool)
    n269 = Index Array(array="Phase input") -> (element=w373:fxp<+,64,64>)  [unwired: 1 in]
    n270 = xnode ("Register Read")() -> ("Data"=w366:u32)  [unwired: 1 in, 1 out]
    n271 = xnode ("Register Read")() -> ("Data"=w368:u16)  [unwired: 1 in, 1 out]
    n272 = feedback #27() -> (w372:fxp<+,64,64>)  [unwired: 1 in]
    n273 = feedback-in #27(w373) -> ()
    n274 = call "SignalGenerator.vi"("phase"=w372, "Reset"=w367) -> ("Cos"=w377:fxp<+/-,16,0>, "Sin"=w376:fxp<+/-,16,0>)  [unwired: 7 in, 1 out]
    n275 = case shown="True" w375 {
      tunnel: w382 -> [_ w396]
      tunnel: w380 -> [_ w395]
      tunnel: w377 -> [_ w389]
      tunnel: w376 -> [_ w388]
      tunnel: w368 -> [_ w387]
      tunnel: w367 -> [_ w386]
      tunnel: w366 -> [_ w385]
      frame False {
      }
      frame True {
        n276 = call "MixAndDownsample_5782_10MhzPID.vi"("Count to skip"=w385, "reset"=w386, "sin0"=w388, "factor"=w387, "cos0"=w389, "signal 0"=w396) -> ("data valid"=w392:bool, "Q out"=w393:fxp<+/-,32,14>, "I out"=w394:fxp<+/-,32,14>)  [unwired: 3 in]
        n277 = call "MixAndDownsample_5782_10MhzPID.vi"("Count to skip"=w385, "reset"=w386, "sin0"=w388, "factor"=w387, "cos0"=w389, "signal 0"=w395) -> ("Q out"=w390:fxp<+/-,32,14>, "I out"=w391:fxp<+/-,32,14>)  [unwired: 3 in, 1 out]
        n278 = case shown="True" w392 {
          tunnel: w393 -> [_ w400]
          tunnel: w394 -> [_ w401]
          tunnel: w391 -> [_ w399]
          tunnel: w390 -> [_ w398]
          frame False {
          }
          frame True {
            n279 = Build Array(w401, w400, w399, w398) -> (w402:fxp<+/-,32,14>[])
            n280 = xnode ("FIFO Method Node")("Element"=w402, "Timeout"=0) -> ()  [unwired: 1 in, 2 out]
          }
        }
      }
    }
  }
  n281 = timed-loop {
    timing: w11 -> [_]
    timing-out: [_] -> w10
    stop <- _ stop-if-true
    n282 = xnode ("FIFO Method Node")("Timeout"=0) -> ("Element"=w415:u64, "Timed Out?"=w413:bool)  [unwired: 1 in, 1 out]
    n283 = feedback #28() -> (w414:u64)  [unwired: 1 in]
    n284 = feedback-in #28(w415) -> ()
    n285 = feedback #29() -> (w412:bool)  [unwired: 1 in]
    n286 = feedback-in #29(w413) -> ()
    n287 = call "HandleFeedForward.vi"("timed out"=w412, "Value"=w414) -> ()  [unwired: 10 in]
  }
  n288 = timed-loop {
    timing: w9 -> [_]
    timing-out: [_] -> w8
    shift-right: [w420] -> _
    shift-left: FeedForwardState."Wait for trigger" ("FF state") -> [w429]
    shift-right: [w421] -> _
    shift-left: TRUE ("decrement") -> [w422]
    stop <- _ stop-if-true
    n289 = feedback #30() -> (w426:bool)  [unwired: 1 in]
    n290 = call-poly <instrlib>:"Count Down.vi"("count in"=u8 2, "load"=w426, "decrement"=TRUE) -> ("terminal count"=w425:bool)  [unwired: 11 in, 1 out]
    n291 = feedback-in #30(w425) -> ()
    n292 = call "Adress counter.vi"("input valid"=w425, "Reset"=w422) -> ("output valid"=w424:bool, "Address"=w432:u32)  [unwired: 8 in]
    n293 = feedback #31() -> (w431:u32)  [unwired: 1 in]
    n294 = feedback-in #31(w432) -> ()
    n295 = case shown="\"Read FF\"" w429 {
      selector: w429 -> [w439 w451 w470 w485]
      tunnel: w431 -> [_ _ w467 w482]
      tunnel: [w438 w456 w469 w484] -> w420
      tunnel: "Load FF" -> [w449 w455 _ _]
      tunnel: w424 -> [_ _ w459 _]
      tunnel: "Clear feedback buffers" -> [w445 w454 _ _]
      tunnel: [TRUE ("decrement") TRUE ("decrement") _ _] -> w421
      tunnel: "FF buffers manual" -> [w436 _ _ _]
      frame "Wait for trigger", Default {
        n296 = Select(t=FeedForwardState."Read FF" ("FF state"), s=w449, f=w439) -> (s? t:f=w446:T4)
        n297 = xnode ("Register Write")() -> ("Data"=w442:bool)  [unwired: 1 in, 1 out]
        n298 = xnode ("Register Write")() -> ("Data"=w443:bool)  [unwired: 1 in, 1 out]
        n299 = Select(t=FeedForwardState."Clear FF" ("FF state"), s=w445, f=w446) -> (s? t:f=w440:T4)
        n300 = Not(x=w443) -> (.not. x?=w441:bool)
        n301 = And(x=w442, y=w441) -> (x .and. y?=w437:bool)
        n302 = And(x=w436, y=w437) -> (x .and. y?=w435:bool)
        n303 = call <instrlib>:"Detect Rising Edge.vi"("signal"=w437) -> ("edge detected"=w434:bool)  [unwired: 14 in]
        n304 = Or(x=w435, y=w434) -> (x .or. y?=w433:bool)
        n305 = Select(t=w440, s=w433, f=w439) -> (s? t:f=w438:T4)
      }
      frame "Wait for reset" {
        n306 = Or(x=w454, y=w455) -> (x .or. y?=w453:bool)
        n307 = Select(t=w451, s=w453, f=FeedForwardState."Wait for trigger" ("FF state")) -> (s? t:f=w456:T4)
      }
      frame "Read FF" {
        n308 = xnode ("Memory Method Node")("Address"=w467) -> ("Data"=w478:fxp<+/-,32,14>)  [unwired: 1 in, 1 out]
        n309 = xnode ("Memory Method Node")("Address"=w467) -> ("Data"=w479:fxp<+/-,32,14>)  [unwired: 1 in, 1 out]
        n310 = xnode ("Memory Method Node")("Address"=w467) -> ("Data"=w477:fxp<+/-,32,14>)  [unwired: 1 in, 1 out]
        n311 = xnode ("Memory Method Node")("Address"=w467) -> ("Data"=w468:fxp<+/-,32,14>)  [unwired: 1 in, 1 out]
        n312 = xnode ("Memory Method Node")("Address"=w467) -> ("Data"=w476:fxp<+/-,32,14>)  [unwired: 1 in, 1 out]
        n313 = xnode ("Memory Method Node")("Address"=w467) -> ("Data"=w466:fxp<+/-,32,14>)  [unwired: 1 in, 1 out]
        n314 = feedback #32() -> (w475:fxp<+/-,32,14>)  [unwired: 1 in]
        n315 = feedback-in #32(w478) -> ()
        n316 = feedback #33() -> (w474:fxp<+/-,32,14>)  [unwired: 1 in]
        n317 = feedback-in #33(w477) -> ()
        n318 = feedback #34() -> (w465:fxp<+/-,32,14>)  [unwired: 1 in]
        n319 = feedback-in #34(w468) -> ()
        n320 = feedback #35() -> (w473:fxp<+/-,32,14>)  [unwired: 1 in]
        n321 = feedback-in #35(w476) -> ()
        n322 = feedback #36() -> (w464:fxp<+/-,32,14>)  [unwired: 1 in]
        n323 = feedback-in #36(w466) -> ()
        n324 = feedback #37() -> (w462:fxp<+/-,32,14>)  [unwired: 1 in]
        n325 = feedback-in #37(w479) -> ()
        n326 = xnode ("Register Read")() -> ("Data"=w460:u16)  [unwired: 1 in, 1 out]
        n327 = Build Array(w462, w475, w474, w473, w465, w464) -> (w461:fxp<+/-,32,14>[])
        n328 = call "FormatDMAelement_6_elements.vi"("valid in"=w459, "factor"=w460, "Data in"=w461) -> ("valid out"=w457:bool, "Values"=w458:u64[])  [unwired: 7 in]
        n329 = case shown="True" w457 {
          tunnel: w458 -> [_ w480]
          frame False {
          }
          frame True {
            n330 = xnode ("FIFO Method Node")("Element"=w480, "Timeout"=0) -> ()  [unwired: 1 in, 2 out]
          }
        }
        n331 = Less?(x=w467, y=u32 40000) -> (x < y?=w471:bool)
        n332 = Select(t=w470, s=w471, f=FeedForwardState."Wait for reset" ("FF state")) -> (s? t:f=w469:T4)
        "Read FF address" <- w467
      }
      frame "Clear FF" {
        w483 = fxp<+/-,32,14> 0.0 ("Data")
        n333 = xnode ("Memory Method Node")("Address"=w482, "Data"=w483) -> ()  [unwired: 1 in, 1 out]
        n334 = xnode ("Memory Method Node")("Address"=w482, "Data"=w483) -> ()  [unwired: 1 in, 1 out]
        n335 = xnode ("Memory Method Node")("Address"=w482, "Data"=w483) -> ()  [unwired: 1 in, 1 out]
        n336 = xnode ("Memory Method Node")("Address"=w482, "Data"=w483) -> ()  [unwired: 1 in, 1 out]
        n337 = Less?(x=w482, y=u32 40000) -> (x < y?=w487:bool)
        n338 = xnode ("Memory Method Node")("Address"=w482, "Data"=w483) -> ()  [unwired: 1 in, 1 out]
        n339 = xnode ("Memory Method Node")("Address"=w482, "Data"=w483) -> ()  [unwired: 1 in, 1 out]
        n340 = Select(t=w485, s=w487, f=FeedForwardState."Wait for reset" ("FF state")) -> (s? t:f=w484:T4)
      }
    }
  }
  n341 = node-c288() -> (w18:T5)  [unwired: 1 in]
  n342 = timed-loop {
    timing: w18 -> [_]
    timing-out: [_] -> w17
    stop <- _ stop-if-true
    n343 = xnode "FPGA I/O Node"("IO Module\\AO Data Sync"="IO Module\\AO Data Sync") -> ()  [unwired: 1 in, 1 out]
  }
  n344 = node-c288() -> (w20:T5)  [unwired: 1 in]
  n345 = timed-loop {
    timing: w20 -> [_]
    timing-out: [_] -> w19
    stop <- _ stop-if-true
    n346 = xnode "FPGA I/O Node"("IO Module\\SPI Device"="IO Module\\SPI Device", "IO Module\\SPI Address"="IO Module\\SPI Address", "IO Module\\SPI Write Data"="IO Module\\SPI Write Data", "IO Module\\SPI Read"="IO Module\\SPI Read", "IO Module\\SPI Write"="IO Module\\SPI Write") -> ("IO Module\\SPI Idle"=→"IO Module\\SPI Idle":bool, "IO Module\\SPI Read Data"=→"IO Module\\SPI Read Data":u8)  [unwired: 7 in, 7 out]
  }
  n347 = node-c288(w28) -> ()
  n348 = node-c288(w21) -> ()
  n349 = node-c288(w23) -> ()
  n350 = node-c288(w10) -> ()
  n351 = node-c288(w26) -> ()
  n352 = node-c288(w4) -> ()
  n353 = node-c288(w8) -> ()
  n354 = node-c288(w1) -> ()
  n355 = node-c288(w17) -> ()
  n356 = node-c288(w13) -> ()
  n357 = node-c288(w19) -> ()
  n358 = node-c288(w15) -> ()
